vi "KE622x -- Check For Errors.vi"(0 "Resource In":refnum<visa-resource-name>, 1 "Check For SCPI Errors? (T)":bool=TRUE, 5 "Turn Off Output If Compliance?":bool=TRUE, 11 "error in (no error)":errorcluster, 12 "Compliance Check Delay (500 ms)":u32=500) -> (4 "Resource Out (dupl)":refnum<visa-resource-name>, 6 "Interlock Tripped?":bool, 8 "Compliance?":bool, 15 "error out":errorcluster)   [LabVIEW 2013, in "Keithly user program.lvlib"]
uses:
  Keithly user program.lvlib
  Typedefs/KE622x -- On Off Control.ctl
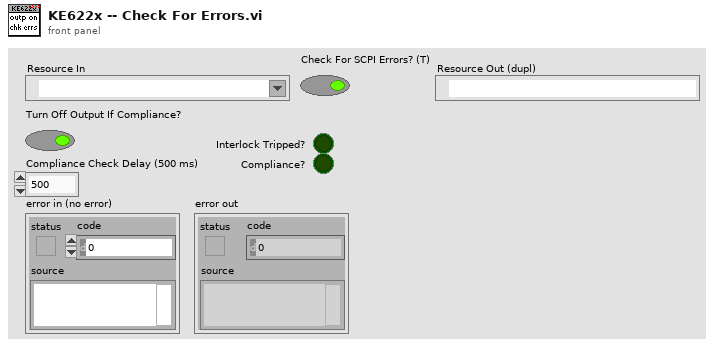
[diagram p1: front panel]
types:
  T1 = typedef "Keithly user program.lvlib/KE622x -- On Off Control.ctl" = enum16{"Off", "On"}
  T2 = typedef "Keithly user program.lvlib/KE622x -- Meas Event Reg State.ctl" = cluster{"B0, ROF:  KE2182A Delta Reading Overflow Event?":bool, "B1, Int:  Interlock OK Event?":bool, "B2, Temp:  Over Temperature Event?":bool, "B3, Comp:  Compliance Event?":bool, "B5, RAV:  Delta Reading Available Event?":bool, "B6, TN:  User Defined Reading Number Stored In Buffer Event?":bool, "B7, BAV:  At Least 2 Readings Stored In Buffer Event?":bool, "B12, BQF:  Buffer Quarter Full Event?":bool, "B8, BHF:  Buffer Half Full Event?":bool, "B13, B3QF:  Buffer 3/4 Full Event?":bool, "B9, BFL:  Buffer Full Event?":bool}
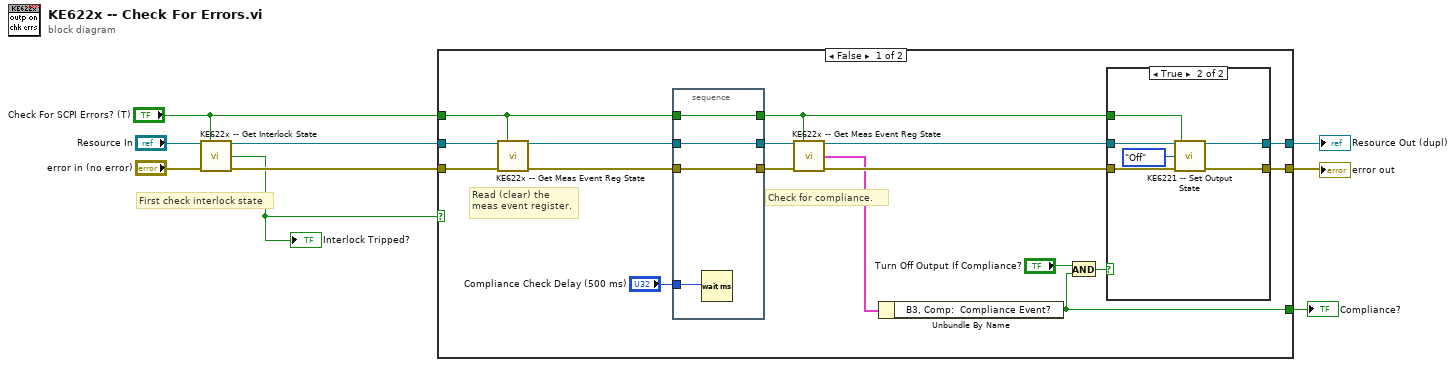
[diagram p0: block diagram]
diagram:
  # "First check interlock state"
  n1 = call "KE622x -- Get Interlock State.vi"("Resource In"="Resource In", "Check For SCPI Errors? (T)"="Check For SCPI Errors? (T)", "error in (no error)"="error in (no error)") -> ("Resource Out (dupl)"=w6:refnum<visa-resource-name>, "Interlock Tripped?"=w2:bool, "error out"=w3:errorcluster)  [unwired: 10 in]
  "Interlock Tripped?" <- w2
  n2 = case shown="False" w2 {
    tunnel: w3 -> [w19 w39]
    tunnel: w6 -> [w20 w40]
    tunnel: "Check For SCPI Errors? (T)" -> [w18 _]
    tunnel: [w24 _] -> w9
    tunnel: [w22 w39] -> w7
    tunnel: [w21 w40] -> w8
    frame False {
      # "Read (clear) the\nmeas event register."
      # "Check for compliance."
      n3 = call "KE622x -- Get Meas Event Reg State.vi"("VISA Resource In"=w20, "Error Query (T)?"=w18, "error in (no error)"=w19) -> ("VISA Resource Out (dupl)"=w11:refnum<visa-resource-name>, "error out"=w10:errorcluster)  [unwired: 10 in, 1 out]
      n4 = stacked-sequence {
        tunnel: "Compliance Check Delay (500 ms)" -> [w38]
        tunnel: w11 -> [w37]
        tunnel: w10 -> [w36]
        tunnel: [w37] -> w17
        tunnel: [w36] -> w14
        tunnel: w18 -> [w35]
        tunnel: [w35] -> w15
        frame #0 {
          n5 = Wait (ms)(milliseconds to wait=w38) -> ()  [unwired: 1 out]
        }
      }
      n6 = call "KE622x -- Get Meas Event Reg State.vi"("VISA Resource In"=w17, "Error Query (T)?"=w15, "error in (no error)"=w14) -> ("VISA Resource Out (dupl)"=w16:refnum<visa-resource-name>, "KE622x Meas Event Reg"=w12:T2, "error out"=w13:errorcluster)  [unwired: 10 in]
      n7 = Unbundle By Name(w12) -> ("B3, Comp:  Compliance Event?"=w24:bool)
      n8 = And(x="Turn Off Output If Compliance?", y=w24) -> (x .and. y?=w23:bool)
      n9 = case shown="True" w23 {
        tunnel: w16 -> [w28 w32]
        tunnel: w13 -> [w27 w31]
        tunnel: w15 -> [_ w30]
        tunnel: [w27 w33] -> w22
        tunnel: [w28 w34] -> w21
        frame False {
        }
        frame True {
          n10 = call "KE6221 -- Set Output State.vi"("Resource In"=w32, "Check For SCPI Errors? (T)"=w30, "Output State"=KE622x_--_On_Off_Control."Off", "error in (no error)"=w31) -> ("Resource Out (dupl)"=w34:refnum<visa-resource-name>, "error out"=w33:errorcluster)  [unwired: 10 in]
        }
      }
    }
    frame True {
    }
  }
  "Resource Out (dupl)" <- w8
  "error out" <- w7
  "Compliance?" <- w9
